vi "execute.vi"(8 "error in (no error)":errorcluster, 11 "Order in":refnum<class "Order.lvclass">) -> (0 "error out":errorcluster, 3 "Order out":refnum<class "Order.lvclass">)   [LabVIEW 2017, in "Order.lvclass"]
uses:
  Order.lvclass
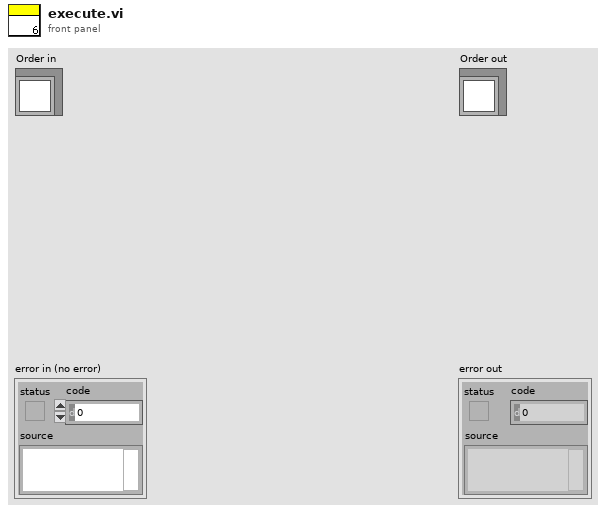
[diagram p1: front panel]
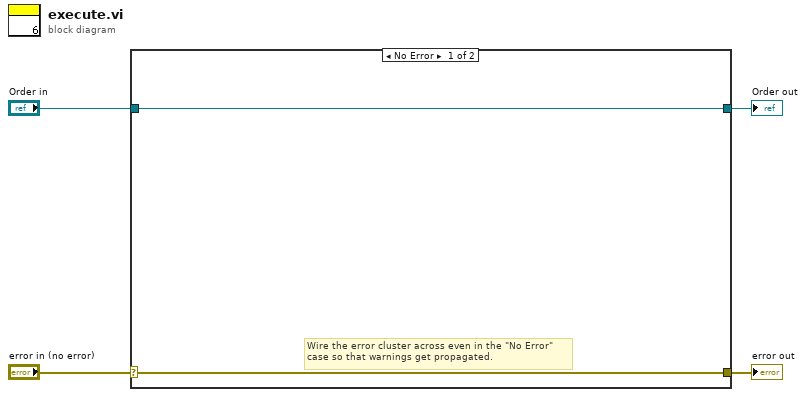
[diagram p0: block diagram]
diagram:
  n1 = case shown="No Error" "error in (no error)" {
    selector: "error in (no error)" -> [w5 w8]
    tunnel: [w5 w8] -> w3
    tunnel: [w6 w7] -> w1
    tunnel: "Order in" -> [w6 w7]
    frame No Error {
      # "Wire the error cluster across even in the \"No Error\"\ncase so that warnings get propagated."
    }
    frame Error {
    }
  }
  "error out" <- w3
  "Order out" <- w1
